vi "Performance Test.vi"() -> ()   [LabVIEW 2021]
uses:
  CIFChannels/Typedef/Direction.ctl
  CIFFifoCAN.lvclass
  ChannelCommon/typedef/FIFO Config.ctl
  <vilib>/Platform/TimedLoop/XDataNode/timing_clust.ctl
  <vilib>/Platform/TimedLoop/XDataNode/nitl_modes.ctl
  <vilib>/Platform/TimedLoop/XDataNode/wakeup.ctl
  ChannelRegistrar/typedef/Datatype CAN.ctl
  CIFCore/Common/Utilities/Add Error.vi
  CIFCore/Common/Utilities/Append Error Location.vi
  <vilib>/Platform/TimedLoop/XDataNode/XDataNode.xnode
  <vilib>/Platform/TimedLoop/XDataNode/XDNodeRunTimeDep.lvlib
  CIFChannels/CIFChannels.lvclass
  ChannelCommon/ChannelCommon.lvlib
  ChannelRegistrar/ChannelRegistrar.lvlib
panel:
  out "timed out?":bool
  out "avg dbl channel":dbl
  out "max dbl channel":dbl
  out "pass":bool
  out "error out":errorcluster
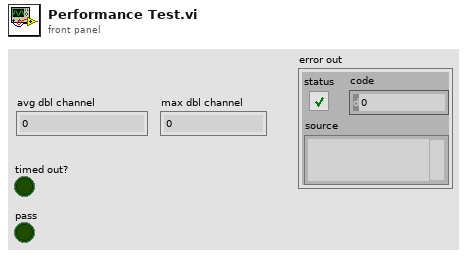
[diagram p1: front panel]
types:
  T1 = typedef "ChannelCommon.lvlib/FIFO Config.ctl" = cluster{"Depth":u64, "Flags":u64}
  T2 = typedef "CIFChannels.lvclass/Direction.ctl" = enum16{"Publisher", "Subscriber"}
  T3 = typedef "ChannelRegistrar.lvlib/Datatype CAN.ctl" = cluster{"payload":u8[], "identifier":u32}
  T4 = typedef "XDNodeRunTimeDep.lvlib/timing_clust.ctl" = cluster{"Expected End [f-1]":u64, "Actual End [f-1]":u64, "Finished Late? [f-1]":bool, "Expected End [i-1]":u64, "Actual End [i-1]":u64, "Finished Late? [i-1]":bool, "Expected Start [i]":u64, "Actual Start [i]":u64, "Expected Start [f]":u64, "Actual Start [f]":u64, "Source Name":string, "Structure Name":string, "Period":i64, "Deadline":i64, "Offset":i64, "Start":i64, "Priority":i32, "Timeout":i32, "Mode":T5, "Wakeup Reason":T6, "Error":errorcluster, "Source Type":string, "Secondary Source Type":string, "Global End Time":u64, "Global Start Time":u64, "Frame Duration":u64, "Iteration Duration":u64, "Assigned CPU":i32, "I/O Scan Engine Mode":u32}
  T5 = typedef "XDNodeRunTimeDep.lvlib/nitl_modes.ctl" = enum32{"No Change", "Process missed periods, maintain original phase", "Discard missed periods, maintain original phase", "Process missed periods, ignore original phase", "Discard missed periods, ignore original phase"}
  T6 = typedef "XDNodeRunTimeDep.lvlib/wakeup.ctl" = enum32{"Normal", "Aborted", "Asynchronous wakeup", "Timing source error", "Timed loop error", "Timeout"}
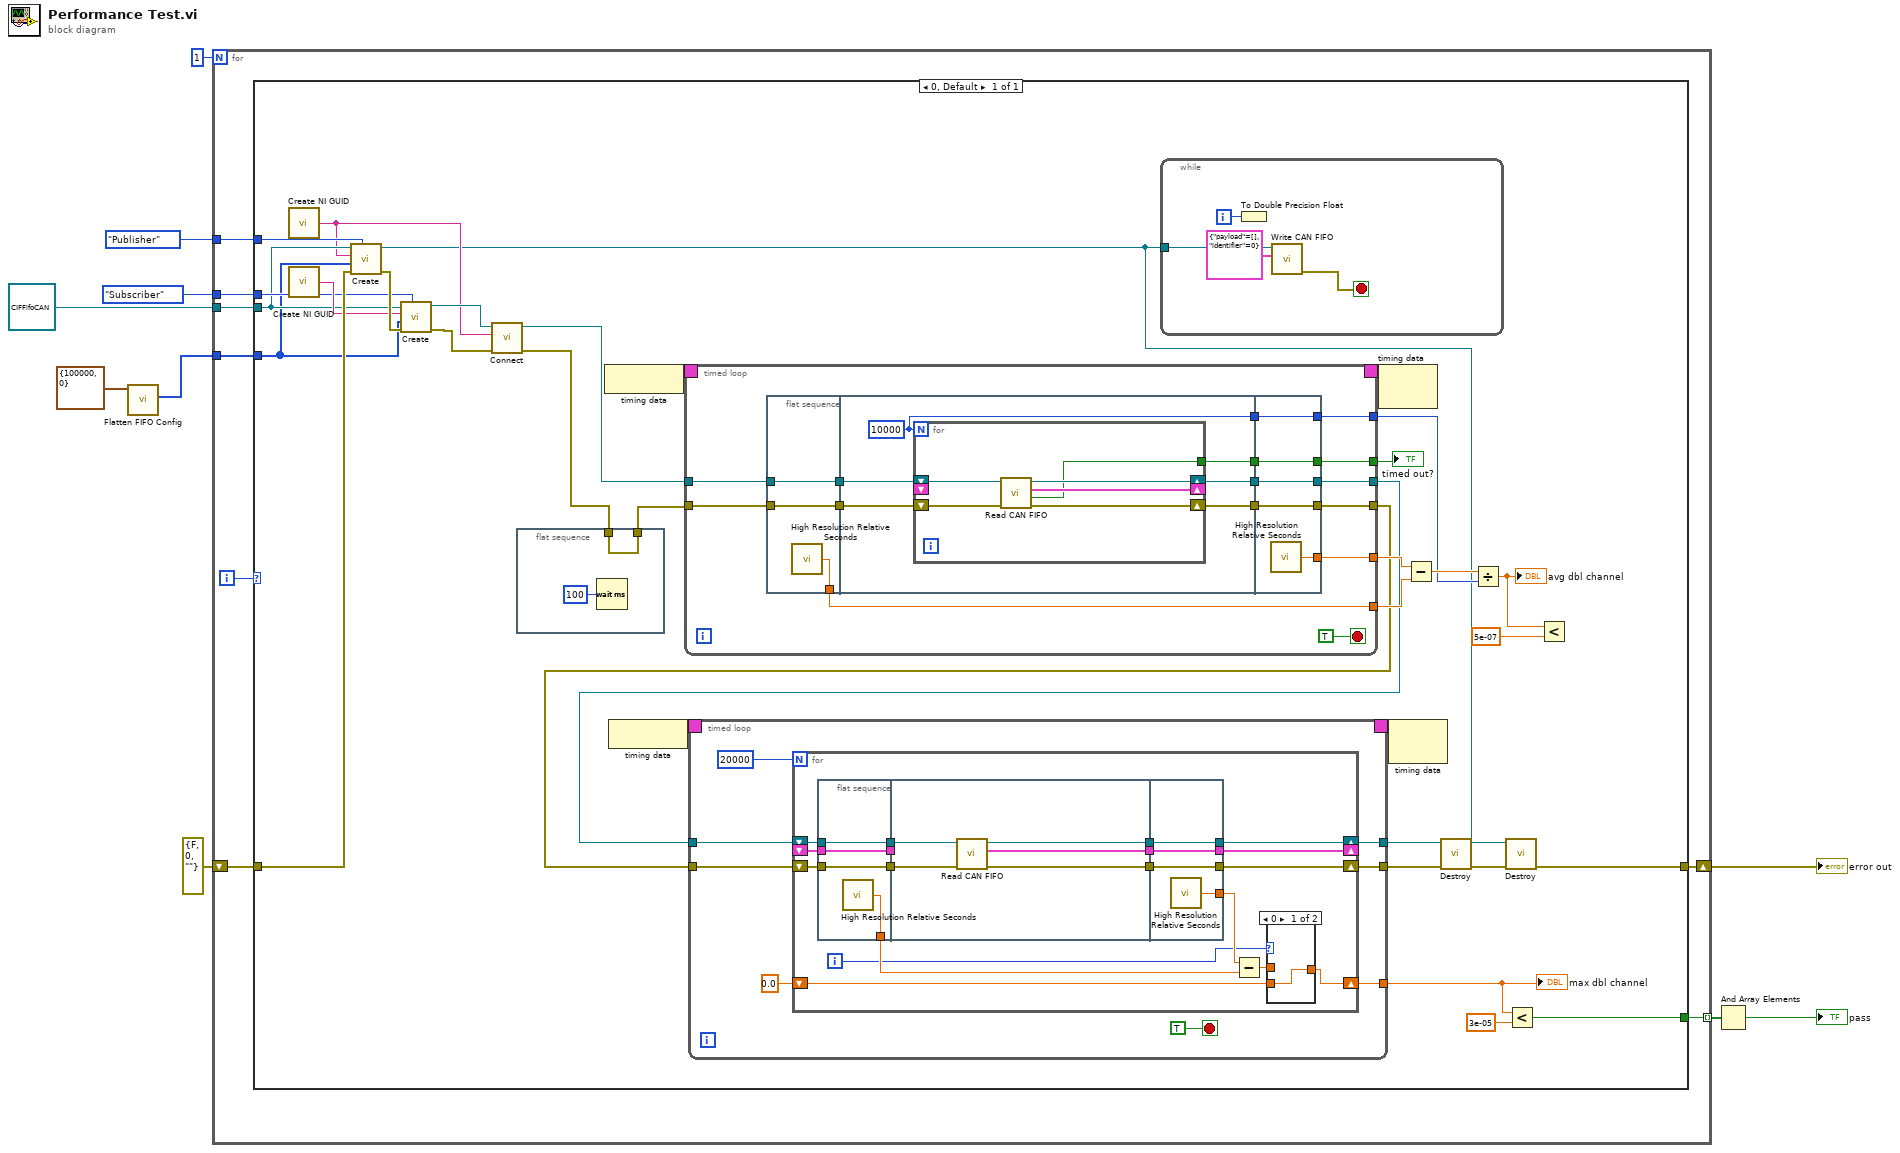
[diagram p0: block diagram]
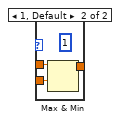
[diagram p2: hidden frame]
diagram:
  n1 = call "Flatten FIFO Config.vi"("FIFO Config in"=T1 {"Depth"=100000, "Flags"=0}) -> ("Flattened Data out"=w2:u8[])  [unwired: 8 in, 2 out]
  n2 = for {
    N: 1 -> [_]
    tunnel: [w18] -> w8 mode=indexing
    shift-right: [w17] -> w10
    shift-left: errorcluster {"status"=FALSE, "code"=0, "source"=""} ("error out") -> [w15]
    tunnel: Direction."Publisher" ("Direction") -> [w14]
    tunnel: Direction."Subscriber" ("Direction") -> [w13]
    tunnel: refnum<class "CIFFifoCAN.lvclass"> refnum ("CIFFifoCAN.lvclass") -> [w12]
    tunnel: w2 -> [w11]
    i -> [w16]
    n3 = case shown="0, Default" w16 {
      tunnel: [w38] -> w18
      tunnel: [w22] -> w17
      tunnel: w15 -> [w36]
      tunnel: w14 -> [w34]
      tunnel: w13 -> [w33]
      tunnel: w12 -> [w32]
      tunnel: w11 -> [w28]
      frame 0, Default {
        n4 = call <vilib>:"Create NI GUID.vi"() -> ("NI GUID"=w30:string)
        n5 = call <vilib>:"Create NI GUID.vi"() -> ("NI GUID"=w35:string)
        n6 = call-dynamic "Create.vi"("Direction"=w34, "error in (no error)"=w36, "Custom Config Data"=w28, "Name"=w30, "CIFTag in"=w32) -> ("error out"=w37:errorcluster, "CIFTag out"=w23:refnum<class "CIFFifoCAN.lvclass">)  [unwired: 5 in]
        n7 = call-dynamic "Create.vi"("Direction"=w33, "error in (no error)"=w37, "Custom Config Data"=w28, "Name"=w35, "CIFTag in"=w32) -> ("error out"=w29:errorcluster, "CIFTag out"=w31:refnum<class "CIFFifoCAN.lvclass">)  [unwired: 5 in]
        n8 = call-dynamic "Connect.vi"("error in (no error)"=w29, "Connection Name"=w30, "CIFTag in"=w31) -> ("error out"=w21:errorcluster, "CIFTag out"=w27:refnum<class "CIFFifoCAN.lvclass">)  [unwired: 7 in]
        n9 = flat-sequence {
          tunnel: w21 -> [w54]
          tunnel: [w54] -> w20
          frame #0 {
            n10 = Wait (ms)(milliseconds to wait=u32 100) -> ()  [unwired: 1 out]
          }
        }
        n11 = node-c288() -> (w52:T4)
        n12 = node-c288() -> (w50:T4)
        n13 = timed-loop {
          timing: w52 -> [_]
          timing-out: [_] -> w51
          tunnel: w27 -> [w120]
          tunnel: w20 -> [w119]
          tunnel: [w115] -> w44
          tunnel: [w113] -> w43
          tunnel: [w111] -> w48
          tunnel: [w110] -> w47
          tunnel: [w109] -> w45
          tunnel: [w107] -> w19
          stop <- TRUE stop-if-true
          n14 = flat-sequence {
            tunnel: w119 -> [w122]
            tunnel: w120 -> [w123]
            tunnel: [w123] -> w117
            tunnel: [w122] -> w116
            tunnel: [w121] -> w110
            tunnel: w117 -> [w129]
            tunnel: w116 -> [w128]
            tunnel: [w127] -> w114
            tunnel: [w126] -> w112
            tunnel: [w125] -> w108
            tunnel: [w124] -> w106
            tunnel: [w140] -> w115
            tunnel: w114 -> [w140]
            tunnel: [w139] -> w113
            tunnel: w112 -> [w139]
            tunnel: [w138] -> w111
            tunnel: [w137] -> w109
            tunnel: w108 -> [w137]
            tunnel: [w136] -> w107
            tunnel: w106 -> [w136]
            frame #0 {
              n15 = call <vilib>:"High Resolution Relative Seconds.vi"() -> ("relative seconds"=w121:dbl)
            }
            frame #1 {
              w125 = 10000
              n16 = for {
                N: w125 -> [_]
                shift-right: [w134] -> w127
                shift-left: w129 -> [w135]
                shift-right: [w132] -> w126
                shift-left: w128 -> [w133]
                shift-right: [w131] -> _
                shift-left: _ -> [_]
                tunnel: [w130] -> w124
                n17 = call-dynamic "Read CAN FIFO.vi"("error in (no error)"=w133, "CIFTag in"=w135) -> ("error out"=w132:errorcluster, "timed out?"=w130:bool, "Data"=w131:T3, "CIFTag out"=w134:refnum<class "CIFFifoCAN.lvclass">)  [unwired: 5 in, 1 out]
              }
            }
            frame #2 {
              n18 = call <vilib>:"High Resolution Relative Seconds.vi"() -> ("relative seconds"=w138:dbl)
            }
          }
        }
        "timed out?" <- w19
        n19 = timed-loop {
          timing: w50 -> [_]
          timing-out: [_] -> w49
          tunnel: w44 -> [w66]
          tunnel: w43 -> [w65]
          tunnel: [w63] -> w26
          tunnel: [w62] -> w25
          tunnel: [w59] -> w40
          stop <- TRUE stop-if-true
          n20 = for {
            N: 20000 -> [_]
            shift-right: [w78] -> w63
            shift-left: w66 -> [w80]
            shift-right: [w77] -> w62
            shift-left: w65 -> [w79]
            shift-right: [w71] -> w59
            shift-left: 0.0 -> [w72]
            shift-right: [w70] -> _
            shift-left: _ -> [w76]
            i -> [w68]
            n21 = flat-sequence {
              tunnel: w79 -> [w91]
              tunnel: w80 -> [w92]
              tunnel: [w92] -> w84
              tunnel: [w91] -> w83
              tunnel: [w90] -> w74
              tunnel: w76 -> [w89]
              tunnel: [w89] -> w82
              tunnel: w84 -> [w97]
              tunnel: w83 -> [w95]
              tunnel: [w96] -> w81
              tunnel: w82 -> [_]
              tunnel: [w93] -> w69
              tunnel: [w94] -> w67
              tunnel: [w101] -> w78
              tunnel: w81 -> [w101]
              tunnel: [w100] -> w77
              tunnel: [w99] -> w75
              tunnel: [w98] -> w70
              tunnel: w69 -> [w98]
              tunnel: w67 -> [w100]
              frame #0 {
                n22 = call <vilib>:"High Resolution Relative Seconds.vi"() -> ("relative seconds"=w90:dbl)
              }
              frame #1 {
                n23 = call-dynamic "Read CAN FIFO.vi"("error in (no error)"=w95, "CIFTag in"=w97) -> ("error out"=w94:errorcluster, "Data"=w93:T3, "CIFTag out"=w96:refnum<class "CIFFifoCAN.lvclass">)  [unwired: 5 in, 2 out]
              }
              frame #2 {
                n24 = call <vilib>:"High Resolution Relative Seconds.vi"() -> ("relative seconds"=w99:dbl)
              }
            }
            n25 = Subtract(x=w75, y=w74) -> (x-y=w73:dbl)
            n26 = case shown="0" w68 {
              tunnel: w73 -> [_ w88]
              tunnel: w72 -> [w85 w87]
              tunnel: [w85 w86] -> w71
              frame 0 {
              }
              frame 1, Default {
                (unwired) u32 1 ("milliseconds to wait")
                n27 = Max & Min(x=w88, y=w87) -> (max(x,y)=w86:dbl)  [unwired: 1 out]
              }
            }
          }
        }
        "max dbl channel" <- w40
        n28 = while {
          tunnel: w23 -> [w57]
          i -> [w58]
          stop <- w55 stop-if-true
          n29 = To Double Precision Float(number=w58) -> ()  [unwired: 1 out]
          n30 = call-dynamic "Write CAN FIFO.vi"("Data"=T3 {"payload"=[], "identifier"=0}, "CIFTag in"=w57) -> ("error out"=w55:errorcluster)  [unwired: 7 in, 2 out]
        }
        n31 = node-c288(w51) -> ()  [unwired: 1 out]
        n32 = node-c288(w49) -> ()  [unwired: 1 out]
        n33 = Subtract(x=w48, y=w47) -> (x-y=w46:dbl)
        n34 = call-dynamic "Destroy.vi"("error in (no error)"=w25, "CIFTag in"=w26) -> ("error out"=w24:errorcluster)  [unwired: 8 in, 1 out]
        n35 = Divide(x=w46, y=w45) -> (x/y=w42:dbl)
        "avg dbl channel" <- w42
        n36 = call-dynamic "Destroy.vi"("error in (no error)"=w24, "CIFTag in"=w23) -> ("error out"=w22:errorcluster)  [unwired: 8 in, 1 out]
        n37 = Less?(x=w40, y=3e-05) -> (x < y?=w38:bool)
        n38 = Less?(x=w42, y=5e-07) -> ()  [unwired: 1 out]
      }
    }
  }
  "error out" <- w10
  n39 = And Array Elements(Boolean array=w8) -> (logical AND=→"pass":bool)
